vi "testDifferentError.vi"() -> ()   [LabVIEW 2017, in "Assertion.Tests.lvlib" / "AssertErrorCode.lvlib"]
uses:
  AssertErrorCode.lvlib
  <vilib>/Utility/error.llb/Error Cluster From Error Code.vi
  <vilib>/ErrorRing/Error Ring.xnode
  Assertion/Assertion.lvlib
panel:
  out "error out":errorcluster
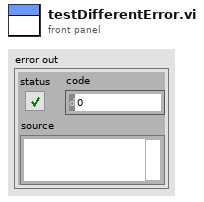
[diagram p1: front panel]
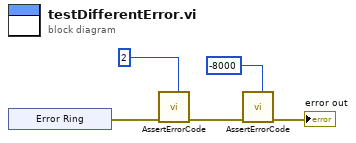
[diagram p0: block diagram]
diagram:
  n1 = xnode "Error Ring"() -> ("error out"=w3:errorcluster)
  n2 = call "AssertErrorCode.vi"("Expected"=2, "error in (no error)"=w3) -> ("error out"=w5:errorcluster)  [unwired: 9 in]
  n3 = call "AssertErrorCode.vi"("Expected"=-8000, "error in (no error)"=w5) -> ("error out"=→"error out":errorcluster)  [unwired: 9 in]
